vi "Gyroscope.vi"() -> (0 "Error Out":errorcluster)   [LabVIEW 2017]
uses:
  <vilib>/myRIO/Instrument Drivers/Onboard IO/I2C/typedefs/I2C User Configuration.ctl
  <vilib>/myRIO/Instrument Drivers/Onboard IO/I2C/typedefs/I2C Transfer Rate.ctl
  <vilib>/Platform/TimedLoop/XDataNode/timing_clust.ctl
  <vilib>/Platform/TimedLoop/XDataNode/nitl_modes.ctl
  <vilib>/Platform/TimedLoop/XDataNode/wakeup.ctl
  <vilib>/myRIO/Common/Instrument Driver Framework/myRIO v1.0/DIO/vis/myRIO v1.1 Open DIO.vi
  <vilib>/myRIO/Common/Instrument Driver Framework/myRIO v1.0/I2C/vis/myRIO v1.1 Open I2C.vi
  <vilib>/myRIO/Common/Instrument Driver Framework/Utilities/vis/Validate Channels.vi
  <vilib>/myRIO/Common/Instrument Driver Framework/myRIO v1.0/DIO/vis/myRIO v1.0 Reserve DIO.vi
  <vilib>/myRIO/Common/Instrument Driver Framework/myRIO v1.0/I2C/vis/myRIO v1.0 Reserve I2C.vi
  <vilib>/myRIO/Common/Instrument Driver Framework/myRIO v1.0/Resource Manager/vis/myRIO v1.0 Reserve Channel List.vi
  <vilib>/myRIO/Common/Instrument Driver Framework/myRIO v1.0/DIO/vis/myRIO v1.0 Build MUX Configuration DIO.vi
  <vilib>/myRIO/Common/Instrument Driver Framework/myRIO v1.0/I2C/vis/myRIO v1.0 Build MUX Configuration I2C.vi
  <vilib>/myRIO/Common/Instrument Driver Framework/myRIO v1.0/Resource Manager/vis/myRIO v1.0 Reserve Channel.vi
  <vilib>/myRIO/Common/Instrument Driver Framework/myRIO v1.0/Resource Manager/vis/myRIO v1.0 Unreserve Channel.vi
  <vilib>/myRIO/Common/Instrument Driver Framework/myRIO v1.0/Resource Manager/vis/myRIO v1.0 Create Configuration List.vi
  <vilib>/myRIO/Common/Instrument Driver Framework/myRIO v1.0/Resource Manager/vis/myRIO v1.0 Build Mutex Name.vi
  <vilib>/Utility/VariantDataType/GetNumericInfo.vi
  <vilib>/Utility/error.llb/Error Cluster From Error Code.vi
  <vilib>/myRIO/Common/Instrument Driver Framework/myRIO v1.0/myRIO v1.1 Open.vi
  <vilib>/myRIO/Common/Instrument Driver Framework/Utilities/vis/IO Manager.vi
  <vilib>/myRIO/Common/Instrument Driver Framework/Utilities/vis/Configuration Manager.vi
  <vilib>/myRIO/Common/Instrument Driver Framework/myRIO v1.0/Resource Manager/vis/myRIO v1.0 Configure IO.vi
  <vilib>/myRIO/Common/Instrument Driver Framework/myRIO v1.0/myRIO v1.0 Close.vi
  <vilib>/myRIO/Common/Instrument Driver Framework/myRIO v1.0/I2C/vis/myRIO v1.0 Configure I2C.vi
  <vilib>/myRIO/Common/Instrument Driver Framework/myRIO v1.0/I2C/vis/myRIO v1.0 Write I2C.vi
  <vilib>/myRIO/Common/Instrument Driver Framework/myRIO v1.0/DIO/vis/myRIO v1.0 Read DIO.vi
  <vilib>/myRIO/Common/Instrument Driver Framework/myRIO v1.0/DIO/vis/myRIO v1.0 Write DIO.vi
  <vilib>/myRIO/Common/Instrument Driver Framework/myRIO v1.0/I2C/vis/myRIO v1.0 Read I2C.vi
  <vilib>/Platform/TimedLoop/XDataNode/XDataNode.xnode
  <vilib>/myRIO/Instrument Drivers/Onboard IO/I2C/I2C.lvlib
  <vilib>/myRIO/Instrument Drivers/Onboard IO/DIO/DIO.lvlib
  <vilib>/Platform/TimedLoop/XDataNode/XDNodeRunTimeDep.lvlib
  <vilib>/ptbypt/NI_PtbyPt.lvlib
panel:
  out "Z (deg per sec)":dbl
  out "CMA (n+1) for Z-Axis Data":dbl
  in  "reset integrator":bool
  out "Z (relative angular displacement)":dbl format="%#_5g"
  out "Y displacement":dbl format="%#_5g"
  out "X displacement":dbl format="%#_5g"
  out "Angular displacement [LSB]":T1(graph)
  out "Angular rate [LSB/sec]":cluster{i16, i16, i16}(graph)
  out "DATA":u8[](array[numeric]) format="%02x"
  out "Z rate":i16
  out "Y rate":i16
  out "X rate":i16
  # "Gyroscope demo"
  # "OUT_X_L"
  # "OUT_X_H"
  # "OUT_Y_L"
  # "OUT_Y_H"
  # "OUT_Z_L"
  # "OUT_Z_H"
  # "Use the CMA value as omega_0 to correct for 'zero-rate level'"
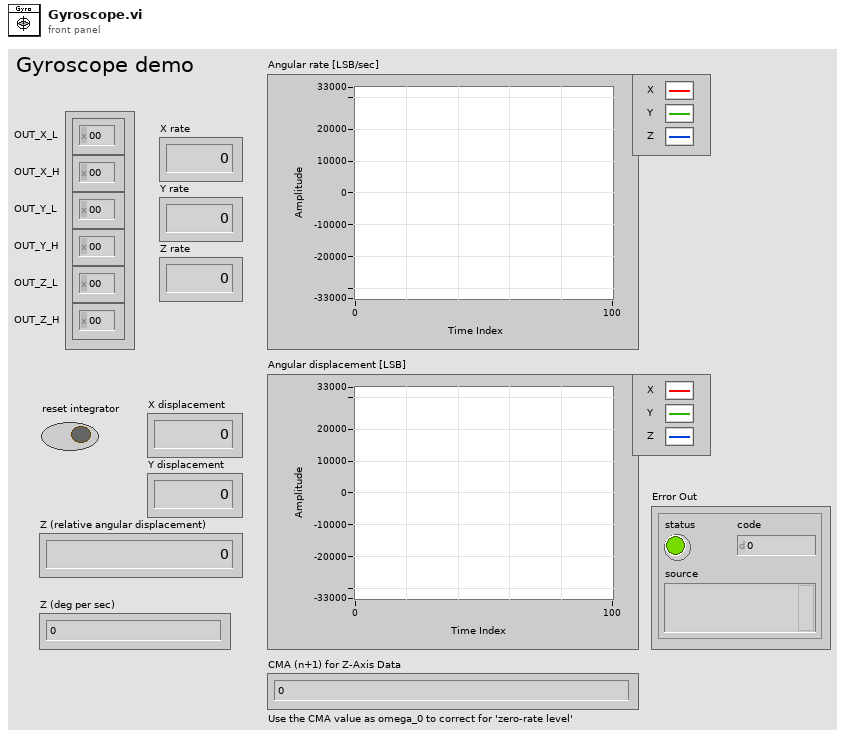
[diagram p1: front panel]
types:
  T1 = cluster{"integral x(t)":dbl, "integral x(t)":dbl, "integral x(t)":dbl}
  T2 = typedef "I2C.lvlib/I2C User Configuration.ctl" = cluster{"I2C Transfer Rate":T3}
  T3 = typedef "I2C.lvlib/I2C Transfer Rate.ctl" = enum16{"Standard mode (100 kbps)", "Fast mode (400 kbps)"}
  T4 = typedef "I2C.lvlib/I2C Reference.ctl" = cluster{"myRIO Reference":T5, "I2C Channels Enum":T9, "I2C Configuration":T10}
  T5 = typedef "myRIO Generic Hardware Reference.ctl" = cluster{"myRIO Model":T6, "myRIO Hardware Reference":T7}
  T6 = typedef "Hardware Version Enum.ctl" = enum16{"Unknown", "myRIO-1900", "myRIO-1950", "roboRIO", "NI ELVIS RIO CM"}
  T7 = typedef "myRIO v1.0 Reference.ctl" = cluster{"Generic FPGA Reference":T8, "Allow multiple opens":bool}
  T8 = typedef "Generic FPGA Reference.ctl" = refnum<k20>
  T9 = typedef "I2C Channels Enum.ctl" = enum16{"Not Connected", "A/I2C", "B/I2C", "I2C/I2C"}
  T10 = typedef "I2C.lvlib/I2C Configuration.ctl" = cluster{"I2C Transfer Rate":T3}
  T11 = typedef "DIO.lvlib/DIO Reference.ctl" = cluster{"myRIO Reference":T5, "DIO Channels List":T12}
  T12 = typedef "DIO Channels List.ctl" = T13[]
  T13 = typedef "DIO Channels Enum.ctl" = enum16{"Not Connected", "C/DIO0", "C/DIO1", "C/DIO2", "C/DIO3", "C/DIO4", "C/DIO5", "C/DIO6", "C/DIO7", "A/DIO0", "A/DIO1", "A/DIO2", "A/DIO3", "A/DIO4", "A/DIO5", "A/DIO6", "A/DIO7", "A/DIO8", "A/DIO9", "A/DIO10", "A/DIO11", "A/DIO12", "A/DIO13", "A/DIO14", "A/DIO15", "B/DIO0", "B/DIO1", "B/DIO2", "B/DIO3", "B/DIO4", "B/DIO5", "B/DIO6", "B/DIO7", "B/DIO8", "B/DIO9", "B/DIO10", "B/DIO11", "B/DIO12", "B/DIO13", "B/DIO14", "B/DIO15", "LED0", "LED1", "LED2", "LED3", "Button0", "DIO/DIO0", "DIO/DIO1", "DIO/DIO2", "DIO/DIO3", "DIO/DIO4", "DIO/DIO5", "DIO/DIO6", "DIO/DIO7", "DIO/DIO8", "DIO/DIO9", "SPI/CS0", "SPI/CS1", "SPI/CS2", "SPI/CS3", "LED RADIO (Green)", "LED RADIO (Red)", "LED COMM (Green)", "LED COMM (Red)", "LED MODE (Green)", "LED MODE (Red)"}
  T14 = typedef "XDNodeRunTimeDep.lvlib/timing_clust.ctl" = cluster{"Expected End [f-1]":u64, "Actual End [f-1]":u64, "Finished Late? [f-1]":bool, "Expected End [i-1]":u64, "Actual End [i-1]":u64, "Finished Late? [i-1]":bool, "Expected Start [i]":u64, "Actual Start [i]":u64, "Expected Start [f]":u64, "Actual Start [f]":u64, "Source Name":string, "Structure Name":string, "Period":i64, "Deadline":i64, "Offset":i64, "Start":i64, "Priority":i32, "Timeout":i32, "Mode":T15, "Wakeup Reason":T16, "Error":errorcluster, "Source Type":string, "Secondary Source Type":string, "Global End Time":u64, "Global Start Time":u64, "Frame Duration":u64, "Iteration Duration":u64, "Assigned CPU":i32, "I/O Scan Engine Mode":u32}
  T15 = typedef "XDNodeRunTimeDep.lvlib/nitl_modes.ctl" = enum32{"No Change", "Process missed periods, maintain original phase", "Discard missed periods, maintain original phase", "Process missed periods, ignore original phase", "Discard missed periods, ignore original phase"}
  T16 = typedef "XDNodeRunTimeDep.lvlib/wakeup.ctl" = enum32{"Normal", "Aborted", "Asynchronous wakeup", "Timing source error", "Timed loop error", "Timeout"}
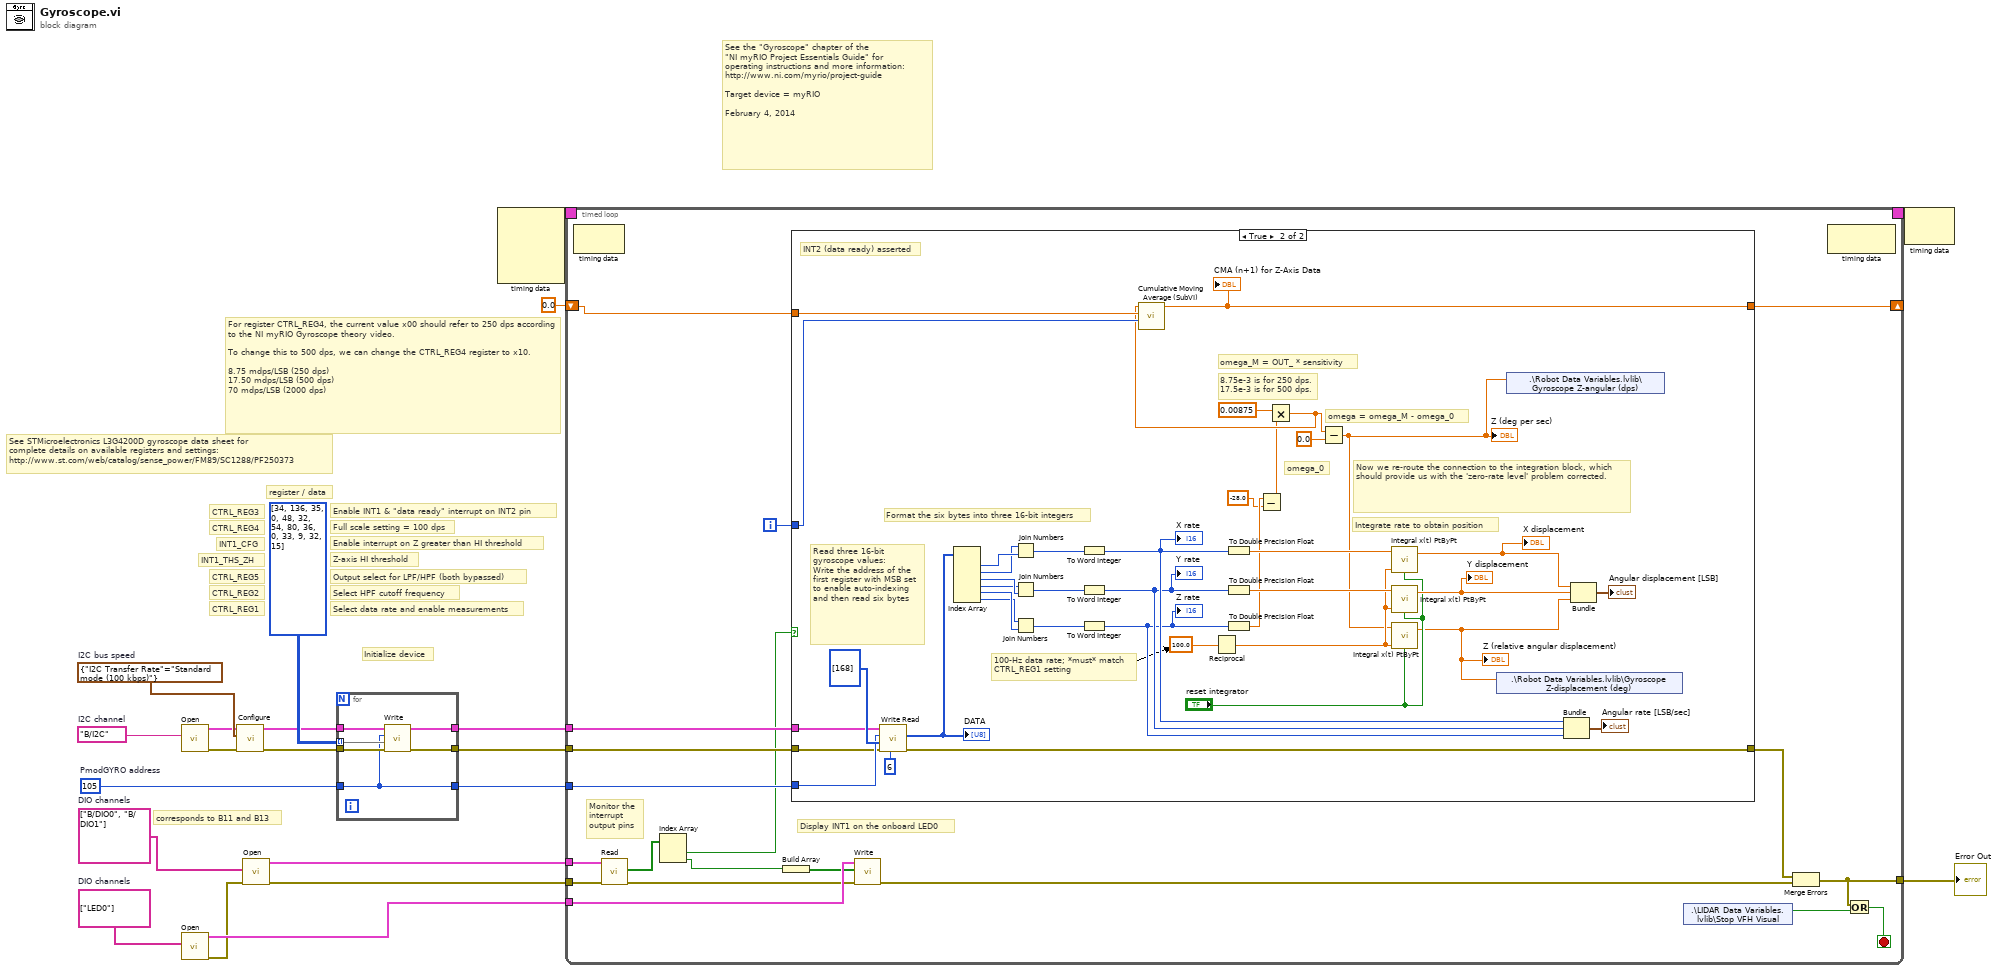
[diagram p0: block diagram]
diagram:
  w5 = tag[] ["LED0"]  # DIO channels
  w8 = tag[] ["B/DIO0", "B/DIO1"]  # DIO channels
  w20 = T2 {"I2C Transfer Rate"=enum."Standard mode (100 kbps)"}  # I2C bus speed
  w21 = tag "B/I2C"  # I2C channel
  w11 = u8 105  # PmodGYRO address
  # "corresponds to B11 and B13"
  # "For register CTRL_REG4, the current value x00 should refer to 250 dps according to the NI myRIO Gyroscope theory video.\n\nTo change this to 500 dps, we can change the CTRL_REG4 register to x10.\n\n8.75 mdps/LSB (250 dps)\n17.50 mdps/LSB (500 dps)\n70 mdps/LSB (2000 dps)"
  # "See the \"Gyroscope\" chapter of the\n\"NI myRIO Project Essentials Guide\" for\noperating instructions and more information: \nhttp://www.ni.com/myrio/project-guide\n\nTarget device = myRIO\n\nFebruary 4, 2014"
  # "Enable INT1 & \"data ready\" interrupt on INT2 pin"
  # "CTRL_REG3"
  # "Select HPF cutoff frequency"
  # "CTRL_REG2"
  # "Output select for LPF/HPF (both bypassed)"
  # "CTRL_REG5"
  # "Initialize device"
  # "Select data rate and enable measurements"
  # "Z-axis HI threshold"
  # "Enable interrupt on Z greater than HI threshold"
  # "See STMicroelectronics L3G4200D gyroscope data sheet for\ncomplete details on available registers and settings:\nhttp://www.st.com/web/catalog/sense_power/FM89/SC1288/PF250373"
  # "CTRL_REG1"
  # "INT1_THS_ZH"
  # "INT1_CFG"
  # "Full scale setting = 100 dps"
  # "CTRL_REG4"
  # "register / data"
  n1 = call <vilib>:"Open.vi"("Channel Name"=w21) -> ("error out"=w18:errorcluster, "I2C Ref Out"=w19:T4)  [unwired: 9 in]
  n2 = call <vilib>:"Open.vi"("Channel Names"=w5) -> ("error out"=w3:errorcluster, "DIO Ref Out"=w4:T11)  [unwired: 9 in]
  n3 = call <vilib>:"Configure.vi"("error in (no error)"=w18, "I2C User Configuration"=w20, "I2C Ref In"=w19) -> ("error out"=w12:errorcluster, "I2C Ref Out"=w13:T4)  [unwired: 7 in]
  n4 = call <vilib>:"Open.vi"("error in (no error)"=w3, "Channel Names"=w8) -> ("error out"=w10:errorcluster, "DIO Ref Out"=w9:T11)  [unwired: 8 in]
  n5 = for {
    tunnel: [w27] -> w17
    tunnel: [w26] -> w16
    tunnel: [w22] -> w15
    tunnel: u8[][] [[34, 136], [35, 0], [48, 32], [54, 80], [36, 0], [33, 9], [32, 15]] ("Bytes to Write") -> [w25] mode=indexing
    tunnel: w13 -> [w24]
    tunnel: w12 -> [w23]
    tunnel: w11 -> [w22]
    n6 = call <vilib>:"Write.vi"("error in (no error)"=w23, "Bytes to Write"=w25, "Slave Address (7-bit)"=w22, "I2C Ref In"=w24) -> ("error out"=w27:errorcluster, "I2C Ref Out"=w26:T4)  [unwired: 6 in]
  }
  n7 = node-c288() -> (w7:T14)  [unwired: 4 in]
  n8 = timed-loop {
    tunnel: [w32] -> w1
    tunnel: w15 -> [w43]
    tunnel: w17 -> [w45]
    tunnel: w16 -> [w44]
    tunnel: w10 -> [w42]
    tunnel: w9 -> [w41]
    timing: w7 -> [_]
    timing-out: [_] -> w6
    tunnel: w4 -> [w37]
    shift-right: [w31] -> _
    shift-left: 0.0 ("CMA (n+1)") -> [w30]
    i -> [w29]
    stop <- w46 stop-if-true
    # "Display INT1 on the onboard LED0"
    # "Monitor the\ninterrupt\noutput pins"
    n9 = node-c288() -> ()  [unwired: 1 in, 1 out]
    n10 = call <vilib>:"Read.vi"("error in (no error)"=w42, "DIO Ref In"=w41) -> ("error out"=w36:errorcluster, "Values"=w38:bool[])  [unwired: 7 in, 1 out]
    n11 = Index Array "Index Array"(array=w38) -> (element #1=w39:bool, element #2=w34:bool)  [unwired: 2 in]
    n12 = Build Array "Build Array"(w34) -> (w35:bool[])
    n13 = case shown="True" w39 {
      tunnel: w45 -> [w50 w69]
      tunnel: w44 -> [_ w70]
      tunnel: w43 -> [_ w77]
      tunnel: [w50 w76] -> w40
      tunnel: [w49 w59] -> w31
      tunnel: w30 -> [w49 w58]
      tunnel: w29 -> [_ w57]
      frame False {
        # "INT2 (data ready) deasserted"
      }
      frame True {
        # "Now we re-route the connection to the integration block, which should provide us with the 'zero-rate level' problem corrected."
        # "omega_0"
        # "omega = omega_M - omega_0"
        # "8.75e-3 is for 250 dps.\n17.5e-3 is for 500 dps."
        # "omega_M = OUT_ * sensitivity"
        # "100-Hz data rate; *must* match\nCTRL_REG1 setting"
        # "Integrate rate to obtain position"
        # "INT2 (data ready) asserted"
        # "Read three 16-bit gyroscope values:\nWrite the address of the first register with MSB set to enable auto-indexing and then read six bytes"
        # "Format the six bytes into three 16-bit integers"
        n14 = call <vilib>:"Write Read.vi"("Byte Count"=u32 6, "error in (no error)"=w69, "Bytes to Write"=u8[] [168], "Slave Address (7-bit)"=w77, "I2C Ref In"=w70) -> ("error out"=w76:errorcluster, "Bytes Read"=w75:u8[])  [unwired: 3 in, 1 out]
        "DATA" <- w75
        n15 = Index Array "Index Array"(array=w75) -> (element #1=w85:u8, element #2=w84:u8, element #3=w83:u8, element #4=w82:u8, element #5=w81:u8, element #6=w80:u8)  [unwired: 6 in]
        n16 = Join Numbers(hi=w84, lo=w85) -> ((hi.lo)=w89:u16)
        n17 = Join Numbers(hi=w82, lo=w83) -> ((hi.lo)=w88:u16)
        n18 = Join Numbers(hi=w80, lo=w81) -> ((hi.lo)=w87:u16)
        n19 = To Word Integer(number=w89) -> (16bit integer=w74:i16)
        "X rate" <- w74
        n20 = To Word Integer(number=w88) -> (16bit integer=w71:i16)
        "Y rate" <- w71
        n21 = To Word Integer(number=w87) -> (16bit integer=w60:i16)
        "Z rate" <- w60
        n22 = Reciprocal(x=100.0 ("dt")) -> (1/x=w67:dbl)
        n23 = To Double Precision Float(number=w74) -> (double precision float=w63:dbl)
        n24 = To Double Precision Float(number=w71) -> (double precision float=w73:dbl)
        n25 = To Double Precision Float(number=w60) -> (double precision float=w56:dbl)
        n26 = Subtract(x=w56, y=-28.0 ("x")) -> (x-y=w52:dbl)
        n27 = Multiply(x=0.00875 ("y"), y=w52) -> (x*y=w53:dbl)
        n28 = call "Cumulative Moving Average (SubVI).vi"("(n)"=w57, "CMA (n)"=w58, "x (n+1)"=w53) -> ("CMA (n+1)"=w59:dbl)  [unwired: 8 in]
        "CMA (n+1) for Z-Axis Data" <- w59
        n29 = Subtract(x=w53, y=0.0) -> (x-y=w55:dbl)
        "Z (deg per sec)" <- w55
        n30 = call <vilib>:"Integral x(t) PtByPt.vi"("initialize"="reset integrator", "dt"=w67, "x"=w63) -> ("integral x(t)"=w64:dbl)  [unwired: 1 in, 1 out]
        "X displacement" <- w64
        n31 = call <vilib>:"Integral x(t) PtByPt.vi"("initialize"="reset integrator", "dt"=w67, "x"=w73) -> ("integral x(t)"=w66:dbl)  [unwired: 1 in, 1 out]
        "Y displacement" <- w66
        n32 = call <vilib>:"Integral x(t) PtByPt.vi"("initialize"="reset integrator", "dt"=w67, "x"=w55) -> ("integral x(t)"=w54:dbl)  [unwired: 1 in, 1 out]
        "Z (relative angular displacement)" <- w54
        n33 = shared-variable ".\\Robot Data Variables.lvlib\\Gyroscope Z-displacement (deg)"(w54) -> ()  [unwired: 1 in, 1 out]
        n34 = shared-variable ".\\Robot Data Variables.lvlib\\Gyroscope Z-angular (dps)"(w55) -> ()  [unwired: 1 in, 1 out]
        n35 = Bundle "Bundle"(w74, w71, w60) -> (→"Angular rate [LSB/sec]":cluster{i16, i16, i16})  [unwired: 1 in]
        n36 = Bundle "Bundle"("integral x(t)"=w64, "integral x(t)"=w66, "integral x(t)"=w54) -> (→"Angular displacement [LSB]":T1)  [unwired: 1 in]
      }
    }
    n37 = call <vilib>:"Write.vi"("error in (no error)"=w36, "Values"=w35, "DIO Ref In"=w37) -> ("error out"=w33:errorcluster)  [unwired: 6 in, 1 out]
    n38 = shared-variable ".\\LIDAR Data Variables.lvlib\\Stop VFH Visual"() -> (w28:bool)  [unwired: 1 in, 1 out]
    n39 = Merge Errors "Merge Errors"(w40, w33) -> (w32:errorcluster)
    n40 = node-c288() -> ()  [unwired: 1 in, 1 out]
    n41 = Or(x=w32, y=w28) -> (x .or. y?=w46:bool)
  }
  "Error Out" <- w1
  n42 = node-c288(w6) -> ()  [unwired: 1 out]
